vi "IMAQ FPGA Configure Image Transfer to Target U16.vi"(5 "DMA FIFO Depth in Images":u32=2, 7 "Image Size":T1, 8 "error in (no error)":errorcluster, 9 "Resource Names":T3, 10 "FPGA VI Reference In":refnum<k20>, 11 "Image":T2) -> (0 "error out":errorcluster, 1 "DMA FIFO Reference Out":refnum<k20>, 2 "DMA FIFO Depth in Elements":u32, 3 "Image Out":T2)   [LabVIEW 2017, in "NI_VDM_FPGA_Basics.lvlib"]
doc: "Configures the transfer of an image from the host processor to the target FPGA via a DMA FIFO. If the <B>Image Size</B> control specifies non-zero <B>Width</B> and <B>Height</B> values, then the image referenced by <B>Image</B> will be resized to match those values. Otherwise, the original image size is preserved. The resulting image size will be set to the FPGA VI front panel control that matches the IMAQ FPGA Image Size.ctl typedef. In addition, a reference will be opened to the DMA FIFO that will be used to transfer the image from the host computer to the target FPGA."
uses:
  <vilib>/visionFPGA/NI_VDM_FPGA_Basics.lvlib
  <vilib>/vision/Image Controls.llb/IMAQ Image.ctl
  <vilib>/visionFPGA/Controls/IMAQ FPGA Image Size.ctl
  <vilib>/NI/LVFPGA Adv Session Resources/OpenByNameSubVI.vi
  <vilib>/Utility/error.llb/Error Cluster From Error Code.vi
  <vilib>/rvi/interface/common/niFpgaWaitOnOcc.vi
  <vilib>/rvi/interface/common/dynamic/niFpgaEscapeDelimiterAndNull.vi
  <vilib>/rvi/interface/nirviMethod/nirviMethod.xnode
  <vilib>/NI/LVFPGA Adv Session Resources/OpenByName.xnode
  <vilib>/rvi/errors/niLvFpgaMergeErrorWithErrorCode.vi
  <vilib>/FPGAPlugInAG/Dynamic/niLvFpga_ConfigureFifo_Dynamic.vi
  <vilib>/FPGAPlugInAG/Dynamic/niLvFpga_StartFifo_Dynamic.vi
  <vilib>/NI/LVFPGA Adv Session Resources/LVFPGAAdvSessionResources.lvlib
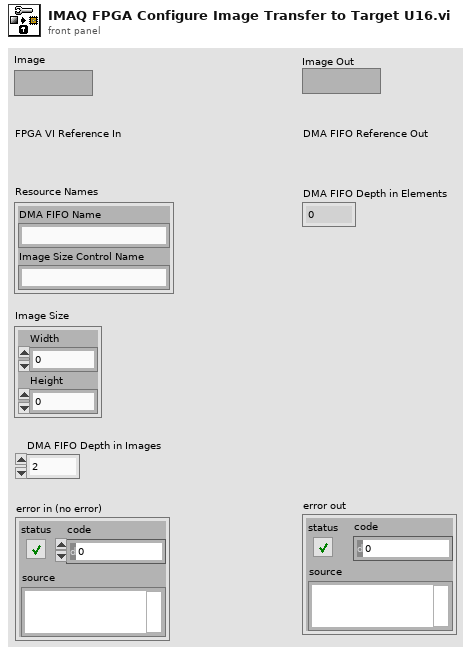
[diagram p1: front panel]
types:
  T1 = typedef "IMAQ FPGA Image Size.ctl" = cluster{"Width":u32, "Height":u32}
  T2 = typedef "IMAQ Image.ctl" = refnum<image>
  T3 = cluster{"DMA FIFO Name":string, "Image Size Control Name":string}
  T4 = cluster{"Name":string, "Depth":u32, "Write? (Deprecated:Use Implementation)":bool, "Physical Channel":u32, "Base Address":u32, "Data Width":u32, "Data Type":enum32{"Boolean", "I8", "I16", "I32", "I64", "U8", "U16", "U32", "U64", "FXP", "CustomControl", "SGL"}, "FXP Properties":variant, "Write Window Address":u32, "Implementation":enum16{"niFpgaTargetToHost", "niFpgaHostToTarget", "niFpgaPeerToPeerWriter", "niFpgaPeerToPeerReader", "niCoreTargetToHost", "niCoreHostToTarget"}, "Control Set":u32}[]
  T5 = cluster{"Name":string, "type":variant, "indicator?":bool}[]
  T6 = typedef "Image Type" = u32
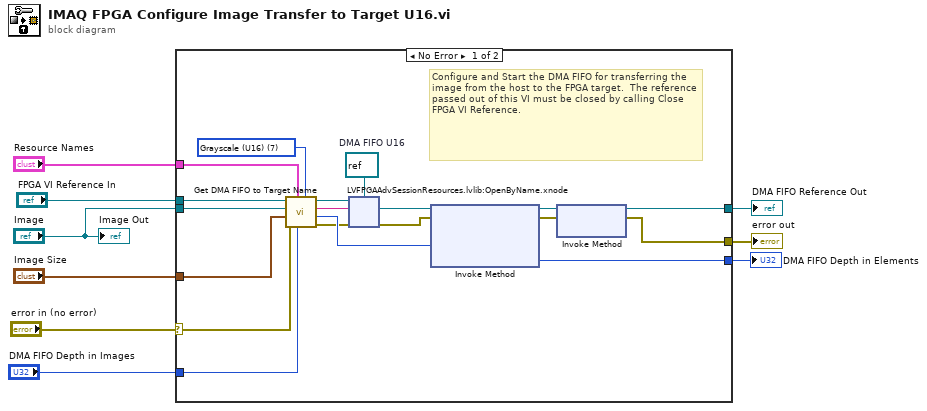
[diagram p0: block diagram]
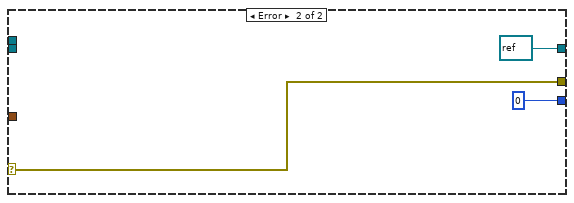
[diagram p2: hidden frame]
diagram:
  n1 = case shown="No Error" "error in (no error)" {
    selector: "error in (no error)" -> [w10 w43]
    tunnel: [w26 w43] -> w9
    tunnel: "Resource Names" -> [w25 _]
    tunnel: "DMA FIFO Depth in Images" -> [w24 _]
    tunnel: "FPGA VI Reference In" -> [w23 _]
    tunnel: "Image Size" -> [w22 _]
    tunnel: "Image" -> [w21 _]
    tunnel: [w19 u32 0 ("Actual Depth")] -> w3
    tunnel: [w17 refnum<k20> refnum ("FPGA VI Reference Out")] -> w2
    frame No Error {
      w16 = refnum<k20> refnum  # DMA FIFO U16
      w18 = T6 7 items=["Grayscale (U8)", "Grayscale (I16)", "Grayscale (SGL)", "Complex (CSG)", "RGB (U32)", "HSL (U32)", "RGB (U64)", "Grayscale (U16)"] ("Image Type")
      # "Configure and Start the DMA FIFO for transferring the image from the host to the FPGA target.  The reference passed out of this VI must be closed by calling Close FPGA VI Reference."
      n2 = call <vilib>:"Get DMA FIFO to Target Name.vi"("Expected Image Type"=w18, "DMA FIFO Depth in Images"=w24, "Resource Names"=w25, "error in (no error)"=w10, "Image Size"=w22, "Image"=w21, "FPGA Refnum In"=w23) -> ("error out"=w13:errorcluster, "DMA FIFO Size"=w20:u32, "DMA FIFO to Target Name"=w14:string, "Refnum out"=w15:refnum<k20>)  [unwired: 1 in]
      n3 = xnode "LVFPGAAdvSessionResources.lvlib:OpenByName.xnode"("FPGA VI Reference in"=w15, "Resource name in"=w14, "Single resource reference type in"=w16, "Error in"=w13) -> ("Single resource reference out"=w12:refnum<k20>, "Error out"=w11:errorcluster)  [unwired: 1 out]
      n4 = xnode "Invoke Method"("FPGA VI Reference In"=w12, "error in"=w11, "Requested Depth"=w20) -> ("FPGA VI Reference Out"=w28:refnum<k20>, "error out"=w27:errorcluster, "Actual Depth"=w19:u32)
      n5 = xnode "Invoke Method"("FPGA VI Reference In"=w28, "error in"=w27) -> ("FPGA VI Reference Out"=w17:refnum<k20>, "error out"=w26:errorcluster)
    }
    frame Error {
    }
  }
  "error out" <- w9
  "DMA FIFO Depth in Elements" <- w3
  "DMA FIFO Reference Out" <- w2
  "Image Out" <- "Image"
